vi "AB_1200_1300_Project_TargetFile_Info.vi"(7 "action":T1, 8 "error in (no error)":errorcluster, 10 "targetfileInfo in":T2, 11 "Object In":T3) -> (0 "error out":errorcluster, 2 "targetfile info":T2, 3 "Object Out":T3)   [LabVIEW 2020]
uses:
  <resource>/Framework/Providers/API/ItemRef.ctl
  <vilib>/AppBuilder/RW_Project/Compatibility/AB_1200_1300_Project_TargetFile_Data.ctl
  <vilib>/AppBuilder/RW_Project/AB_RW_Project_PropBag_Action.ctl
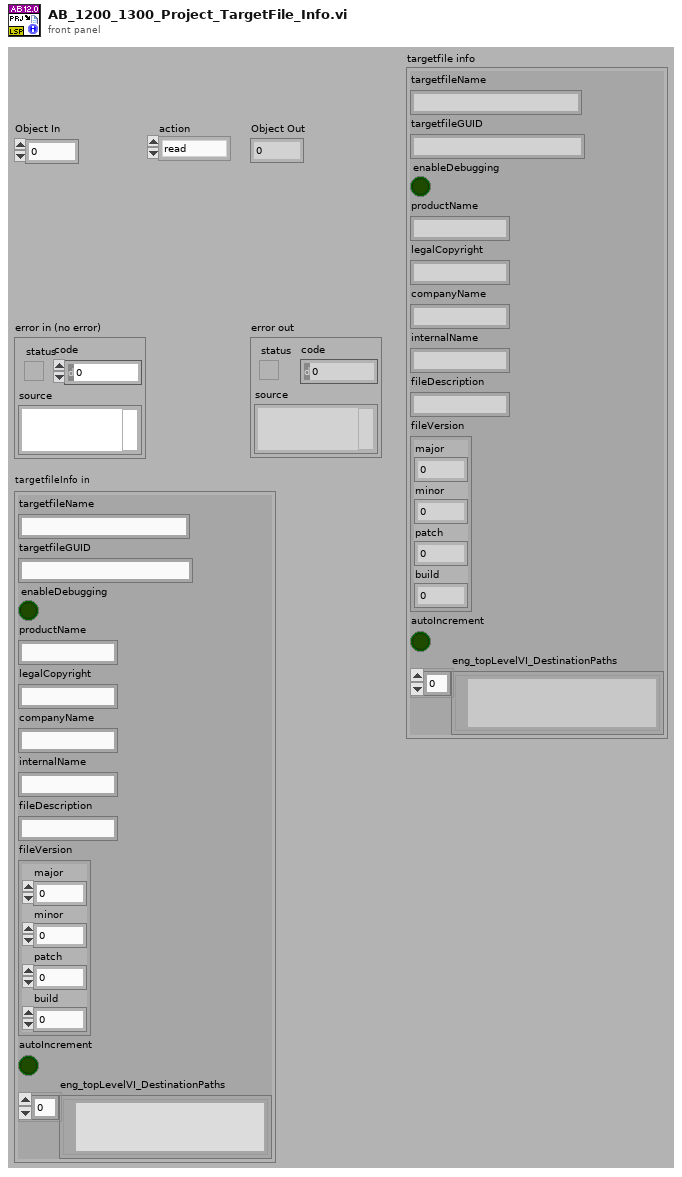
[diagram p1: front panel]
types:
  T1 = typedef "AB_RW_Project_PropBag_Action.ctl" = enum16{"read", "write", "clear", "readPrevious", "writePrevious", "clearPrevious"}
  T2 = typedef "AB_1200_1300_Project_TargetFile_Data.ctl" = cluster{"targetfileName":string, "targetfileGUID":string, "enableDebugging":bool, "productName":string, "legalCopyright":string, "companyName":string, "internalName":string, "fileDescription":string, "fileVersion":cluster{"major":u16, "minor":u16, "patch":u16, "build":u16}, "autoIncrement":bool, "eng_topLevelVI_DestinationPaths":path[]}
  T3 = typedef "ItemRef.ctl" = u64
  T4 = cluster{"[0]":i32, "[1]":i32, "[2]":i32, "[3]":i32}
  T5 = cluster{"major":u16, "minor":u16, "patch":u16, "build":u16}
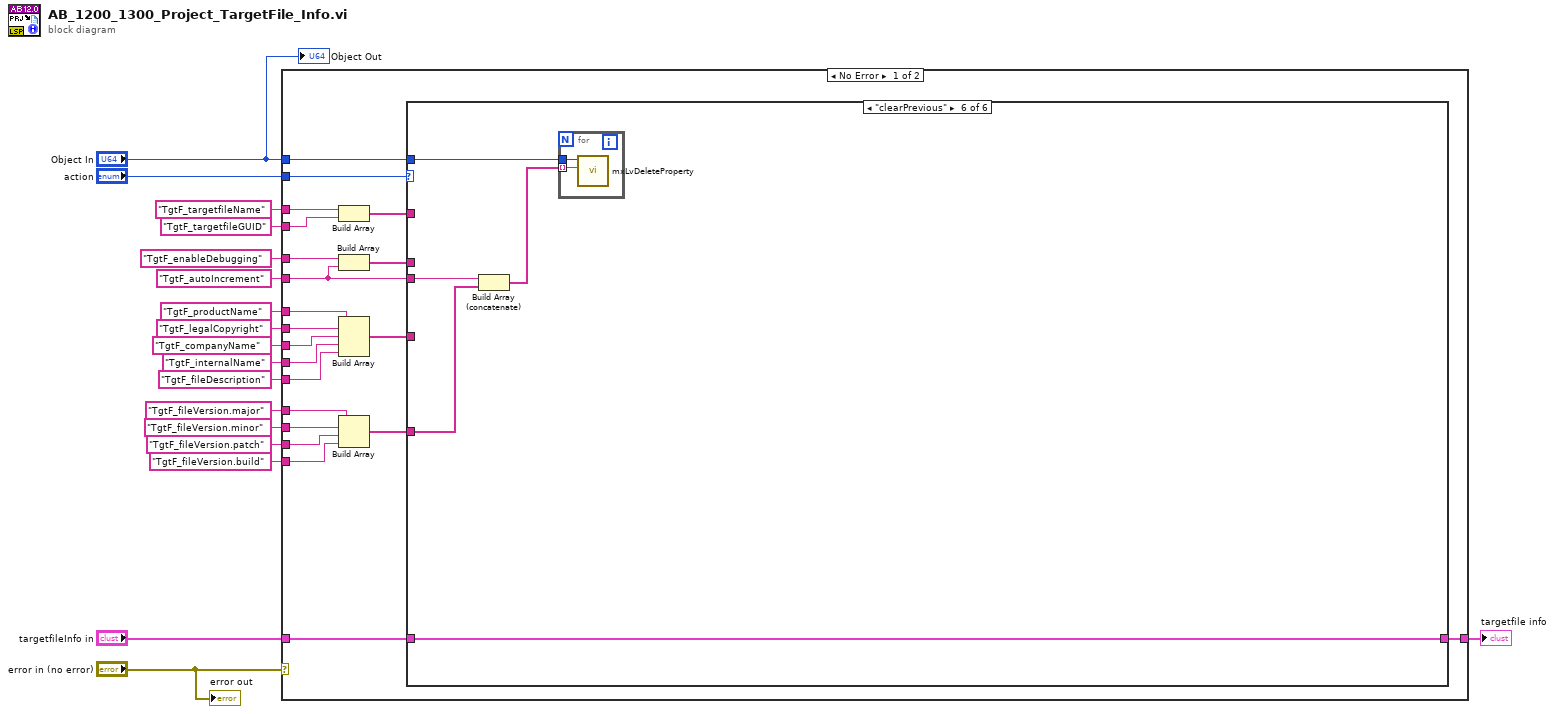
[diagram p0: block diagram]
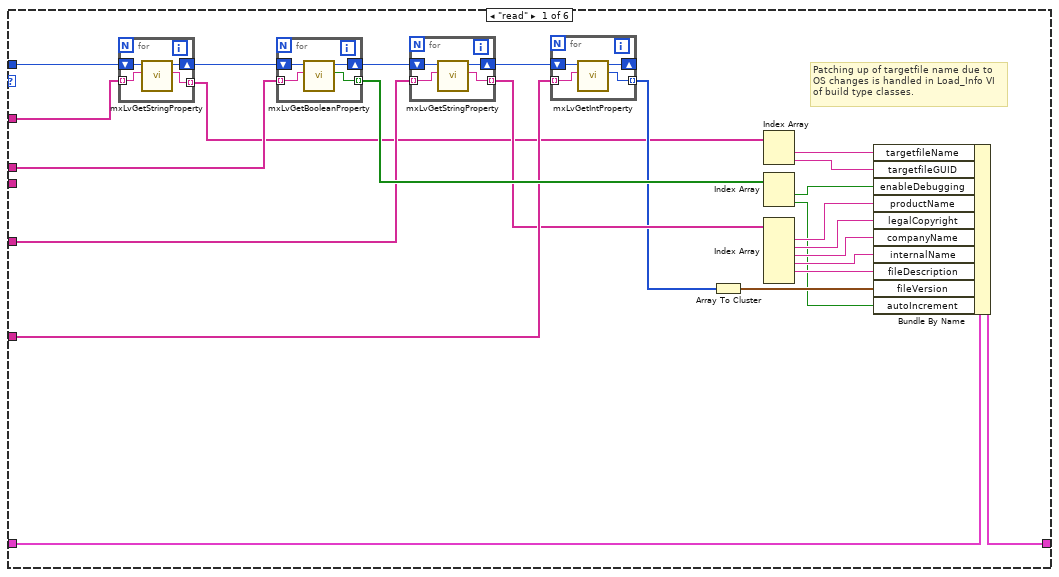
[diagram p2: hidden frame]
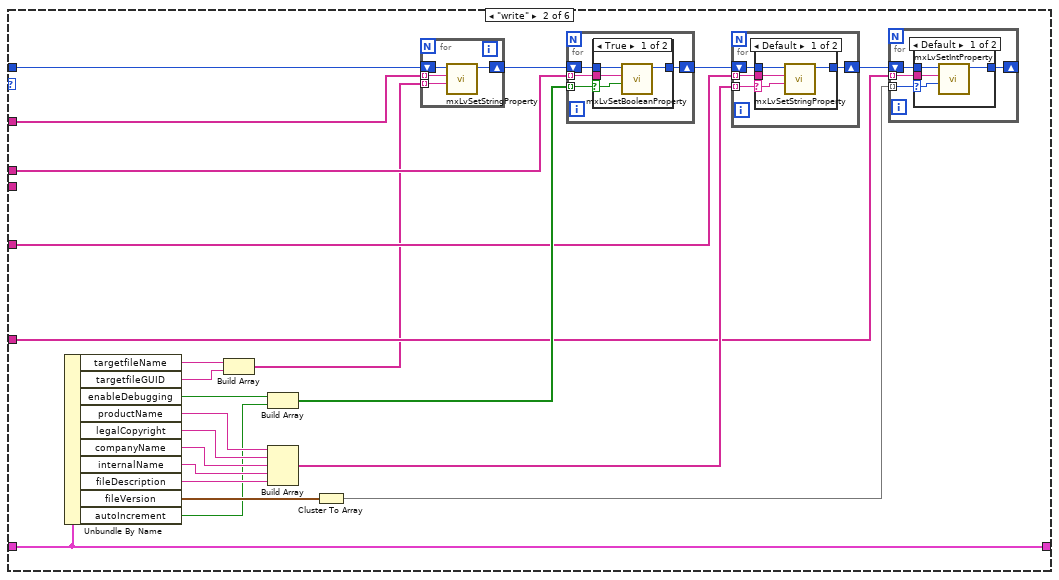
[diagram p3: hidden frame]
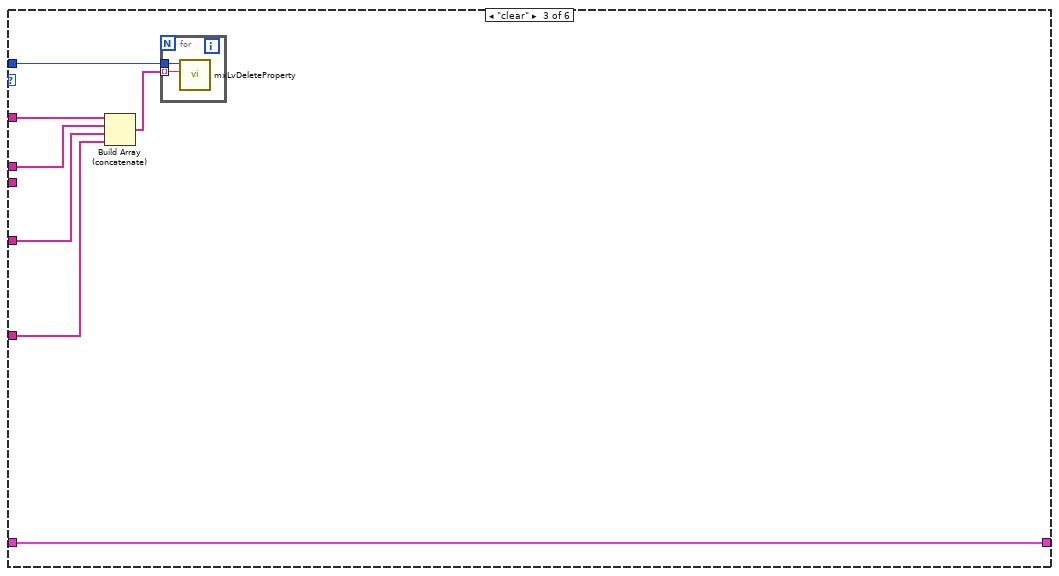
[diagram p7: hidden frame]
diagram:
  n1 = case shown="No Error" "error in (no error)" {
    tunnel: "Object In" -> [w39 _]
    tunnel: [w25 _] -> w16
    tunnel: "targetfileInfo in" -> [w31 _]
    tunnel: "TgtF_targetfileName" ("Tag") -> [w23 _]
    tunnel: "TgtF_enableDebugging" ("Tag") -> [w20 _]
    tunnel: "TgtF_productName" ("Tag") -> [w36 _]
    tunnel: "TgtF_legalCopyright" ("Tag") -> [w37 _]
    tunnel: "TgtF_companyName" ("Tag") -> [w35 _]
    tunnel: "TgtF_internalName" ("Tag") -> [w34 _]
    tunnel: "TgtF_fileDescription" ("Tag") -> [w33 _]
    tunnel: "TgtF_fileVersion.major" ("Tag") -> [w29 _]
    tunnel: "TgtF_fileVersion.minor" ("Tag") -> [w30 _]
    tunnel: "TgtF_fileVersion.patch" ("Tag") -> [w28 _]
    tunnel: "TgtF_fileVersion.build" ("Tag") -> [w27 _]
    tunnel: "TgtF_autoIncrement" ("Tag") -> [w19 _]
    tunnel: "action" -> [w24 _]
    tunnel: "TgtF_targetfileGUID" ("Tag") -> [w22 _]
    frame No Error {
      n2 = Build Array(w23, w22) -> (w21:string[])
      n3 = Build Array(w20, w19) -> (w38:string[])
      n4 = Build Array(w36, w37, w35, w34, w33) -> (w32:string[])
      n5 = Build Array(w29, w30, w28, w27) -> (w26:string[])
      n6 = case shown="\"clearPrevious\"" w24 {
        tunnel: w39 -> [w47 w102 w139 _ _ w146]
        tunnel: w38 -> [w62 w99 w138 _ _ _]
        tunnel: w32 -> [w57 w97 w137 _ _ _]
        tunnel: w31 -> [w63 w80 w140 w143 w144 w149]
        tunnel: w26 -> [w59 w90 w136 _ _ w147]
        tunnel: [w48 w80 w140 w143 w144 w149] -> w25
        tunnel: w21 -> [w46 w85 w134 _ _ _]
        tunnel: w19 -> [_ _ _ _ _ w148]
        frame "read" {
          # "Patching up of targetfile name due to OS changes is handled in Load_Info VI of build type classes."
          n7 = for {
            shift-right: [w66] -> w41
            shift-left: w47 -> [w67]
            tunnel: w46 -> [w64] mode=indexing
            tunnel: [w65] -> w45 mode=indexing
            n8 = call <resource>:"mxLvGetStringProperty.vi"("Tag"=w64, "Item"=w67) -> ("Value"=w65:string, "Item"=w66:T3)  [unwired: 1 in, 7 out]
          }
          n9 = for {
            shift-right: [w78] -> w58
            shift-left: w41 -> [w79]
            tunnel: w62 -> [w77] mode=indexing
            tunnel: [w76] -> w61 mode=indexing
            n10 = call <resource>:"mxLvGetBooleanProperty.vi"("Tag"=w77, "Item"=w79) -> ("Value"=w76:bool, "Item"=w78:T3)  [unwired: 1 in, 7 out]
          }
          n11 = for {
            shift-right: [w74] -> w43
            shift-left: w58 -> [w75]
            tunnel: w57 -> [w72] mode=indexing
            tunnel: [w73] -> w56 mode=indexing
            n12 = call <resource>:"mxLvGetStringProperty.vi"("Tag"=w72, "Item"=w75) -> ("Value"=w73:string, "Item"=w74:T3)  [unwired: 1 in, 7 out]
          }
          n13 = for {
            shift-right: [w70] -> _
            shift-left: w43 -> [w71]
            tunnel: w59 -> [w68] mode=indexing
            tunnel: [w69] -> w50 mode=indexing
            n14 = call <resource>:"mxLvGetIntProperty.vi"("Tag"=w68, "Item"=w71) -> ("Value"=w69:i32, "Item"=w70:T3)  [unwired: 1 in, 7 out]
          }
          n15 = Array To Cluster(array=w50) -> (cluster=w49:T4)
          n16 = Index Array(array=w45) -> (element #1=w42:string, element #2=w44:string)  [unwired: 2 in]
          n17 = Index Array(array=w61) -> (element #1=w60:bool, element #2=w40:bool)  [unwired: 2 in]
          n18 = Index Array(array=w56) -> (element #1=w55:string, element #2=w54:string, element #3=w53:string, element #4=w52:string, element #5=w51:string)  [unwired: 6 in, 1 out]
          n19 = Bundle By Name(cluster=w63, "targetfileName"=w42, "targetfileGUID"=w44, "enableDebugging"=w60, "productName"=w55, "legalCopyright"=w54, "companyName"=w53, "internalName"=w52, "fileDescription"=w51, "fileVersion"=w49, "autoIncrement"=w40) -> (w48:T2)
        }
        frame "write" {
          n20 = Unbundle By Name(w80) -> ("targetfileName"=w84:string, "targetfileGUID"=w83:string, "enableDebugging"=w81:bool, "productName"=w95:string, "legalCopyright"=w96:string, "companyName"=w94:string, "internalName"=w93:string, "fileDescription"=w92:string, "fileVersion"=w89:T5, "autoIncrement"=w86:bool)
          n21 = Build Array(w84, w83) -> (w82:string[])
          n22 = Build Array(w81, w86) -> (w100:bool[])
          n23 = Build Array(w95, w96, w94, w93, w92) -> (w91:string[])
          n24 = Cluster To Array(cluster=w89) -> (array=w88:u16[])
          n25 = for {
            tunnel: w85 -> [w104] mode=indexing
            tunnel: w82 -> [w103] mode=indexing
            shift-right: [w105] -> w101
            shift-left: w102 -> [w106]
            n26 = call <resource>:"mxLvSetStringProperty.vi"("Value (\"\")"=w103, "Tag"=w104, "Item"=w106) -> ("Item"=w105:T3)  [unwired: 2 in, 6 out]
          }
          n27 = for {
            tunnel: w100 -> [w127] mode=indexing
            shift-right: [w126] -> w98
            shift-left: w101 -> [w128]
            tunnel: w99 -> [w125] mode=indexing
            n28 = case shown="True" w127 {
              selector: w127 -> [w131 _]
              tunnel: w128 -> [w132 w133]
              tunnel: w125 -> [w129 _]
              tunnel: [w130 w133] -> w126
              frame True {
                n29 = call <resource>:"mxLvSetBooleanProperty.vi"("Value (F)"=w131, "Tag"=w129, "Item"=w132) -> ("Item"=w130:T3)  [unwired: 2 in, 6 out]
              }
              frame False {
              }
            }
          }
          n30 = for {
            tunnel: w91 -> [w118] mode=indexing
            shift-right: [w117] -> w87
            shift-left: w98 -> [w119]
            tunnel: w97 -> [w116] mode=indexing
            n31 = case shown="Default" w118 {
              selector: w118 -> [w121 _]
              tunnel: w119 -> [w123 w124]
              tunnel: w116 -> [w120 _]
              tunnel: [w122 w124] -> w117
              frame Default {
                n32 = call <resource>:"mxLvSetStringProperty.vi"("Value (\"\")"=w121, "Tag"=w120, "Item"=w123) -> ("Item"=w122:T3)  [unwired: 2 in, 6 out]
              }
              frame "" {
              }
            }
          }
          n33 = for {
            tunnel: w88 -> [w109] mode=indexing
            shift-right: [w108] -> _
            shift-left: w87 -> [w110]
            tunnel: w90 -> [w107] mode=indexing
            n34 = case shown="Default" w109 {
              selector: w109 -> [w113 _]
              tunnel: w110 -> [w114 w115]
              tunnel: w107 -> [w112 _]
              tunnel: [w111 w115] -> w108
              frame Default {
                n35 = call <resource>:"mxLvSetIntProperty.vi"("Value (0)"=w113, "Tag"=w112, "Item"=w114) -> ("Item"=w111:T3)  [unwired: 2 in, 6 out]
              }
              frame 0 {
              }
            }
          }
        }
        frame "clear" {
          n36 = Build Array (concatenate)(w134, w138, w137, w136) -> (w135:string[])
          n37 = for {
            tunnel: w139 -> [w142]
            tunnel: w135 -> [w141] mode=indexing
            n38 = call <resource>:"mxLvDeleteProperty.vi"("Tag"=w141, "Item"=w142) -> ()  [unwired: 1 in, 9 out]
          }
        }
        frame "readPrevious" {
        }
        frame "writePrevious" {
        }
        frame "clearPrevious" {
          n39 = Build Array (concatenate)(w148, w147) -> (w145:string[])
          n40 = for {
            tunnel: w146 -> [w151]
            tunnel: w145 -> [w150] mode=indexing
            n41 = call <resource>:"mxLvDeleteProperty.vi"("Tag"=w150, "Item"=w151) -> ()  [unwired: 1 in, 9 out]
          }
        }
      }
    }
    frame Error {
    }
  }
  "targetfile info" <- w16
  "Object Out" <- "Object In"
  "error out" <- "error in (no error)"
